vi "string_to_byte.vi"(8 "error in (no error)":errorcluster, 10 "Byte (string)":string) -> (0 "error out":errorcluster, 2 "Byte (int)":u8)   [LabVIEW 2018]
doc: "Convert an IC6 response string representing an integer that is 1 byte long into a LabVIEW U8."
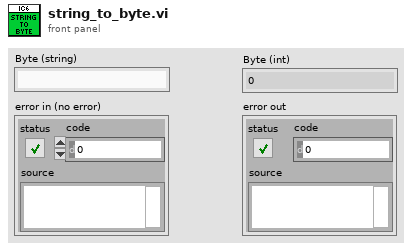
[diagram p1: front panel]
types:
  T1 = enum16{"big-endian, network order", "native, host order", "little-endian"}
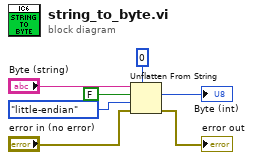
[diagram p0: block diagram]
diagram:
  n1 = Unflatten From String(type=u8 0 ("offset (0)"), binary string="Byte (string)", data includes array or string size? (T)=FALSE, byte order (0:big-endian, network order)=T1."little-endian", error in (no error)="error in (no error)") -> (value=→"Byte (int)":u8, error out=→"error out":errorcluster)  [unwired: 1 out]
